vi "MAIN.vi"() -> ()   [LabVIEW 2012]
uses:
  Control/#TD_ThreadsStates.ctl
  Signal/#TD_SignalStorageCommand.ctl
panel:
  in  "Cancel Button":bool
  in  "Results":bool
  in  "Analysis":bool
  in  "Settings":bool
  in  "Signals":bool
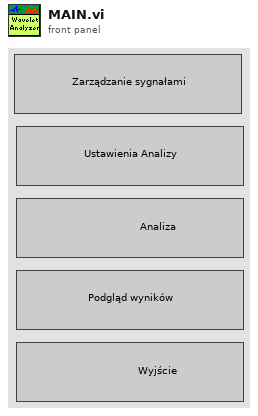
[diagram p1: front panel]
types:
  T1 = typedef "#TD_ThreadsStates.ctl" = cluster{"SigMgmntActive?":bool, "ResltVivActive?":bool, "SettngsMngActive?":bool}
  T2 = typedef "#TD_SignalStorageCommand.ctl" = enum16{"Reset_Storage", "Add_Signal", "Insert_Signal", "Del_Signal", "Replace_Signal", "Get_Signal", "Get_Signal_List", "Change_Signal_Name", "Change_Signal_Descr"}
  T3 = enum32{"Invalid", "Standard", "Closed", "Hidden", "Minimized", "Maximized"}
  T4 = enum32{"Bad", "Idle", "Run top level", "Running"}
  T5 = typedef "#TD_AnalysisSettings.ctl" = cluster{"DecompLevel":i32, "WaveletsToUse":enum16{"db02", "db03", "db04", "db05", "db06", "db07", "db08", "db09", "db10", "db11", "db12", "db13", "db14", "Haar", "bior1_3", "bior1_5", "bior2_2", "bior2_4", "bior2_6", "bior2_8", "bior3_1", "bior3_3", "bior3_5", "bior3_7", "bior3_9", "bior4_4 (FBI)", "bior5_5", "bior6_8", "coif1", "coif2", "coif3", "coif4", "coif5", "sym2", "sym3", "sym4", "sym5", "sym6", "sym7", "sym8"}[], "SignalToAnalysisNb":i32}
  T6 = enum16{"db02", "db03", "db04", "db05", "db06", "db07", "db08", "db09", "db10", "db11", "db12", "db13", "db14", "Haar", "bior1_3", "bior1_5", "bior2_2", "bior2_4", "bior2_6", "bior2_8", "bior3_1", "bior3_3", "bior3_5", "bior3_7", "bior3_9", "bior4_4 (FBI)", "bior5_5", "bior6_8", "coif1", "coif2", "coif3", "coif4", "coif5", "sym2", "sym3", "sym4", "sym5", "sym6", "sym7", "sym8"}[]
  T7 = typedef "#TD_SignalStorageData.ctl" = cluster{"Signal Name":string, "Signal":waveform(dbl), "Description":string}
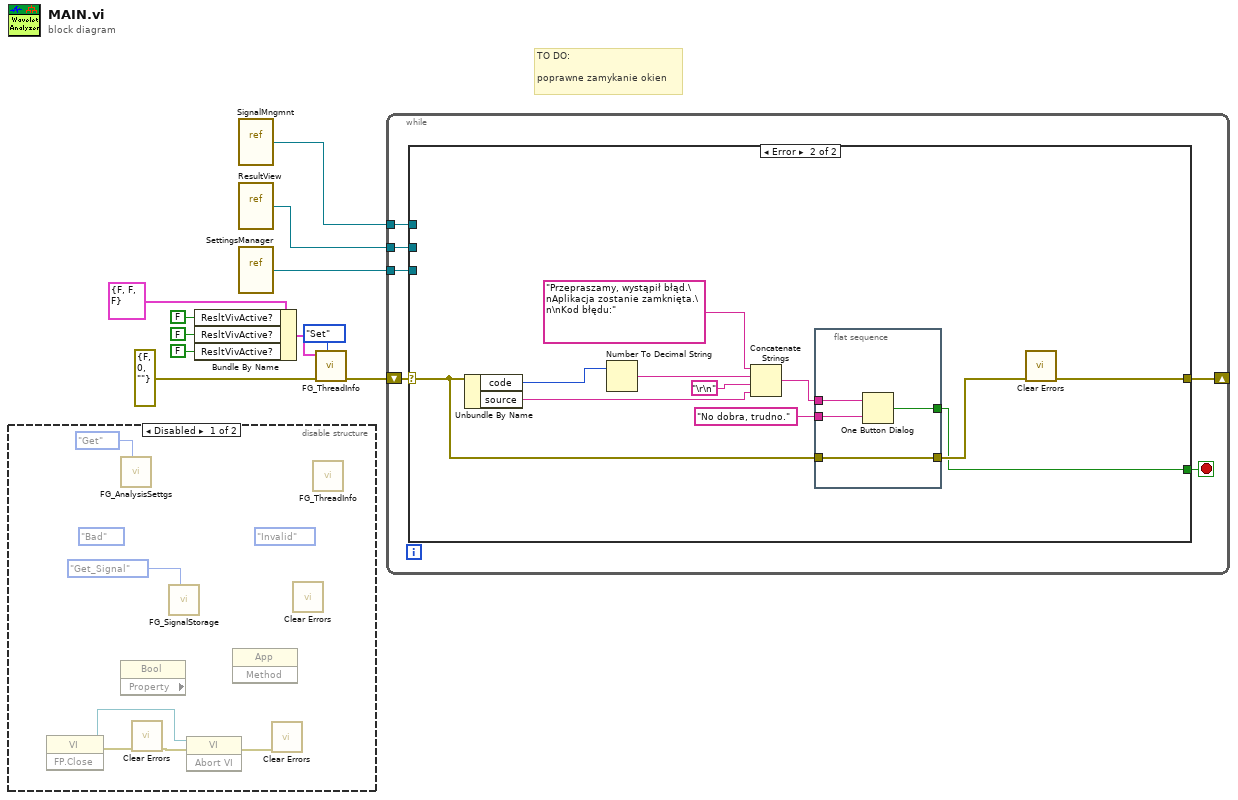
[diagram p0: block diagram]
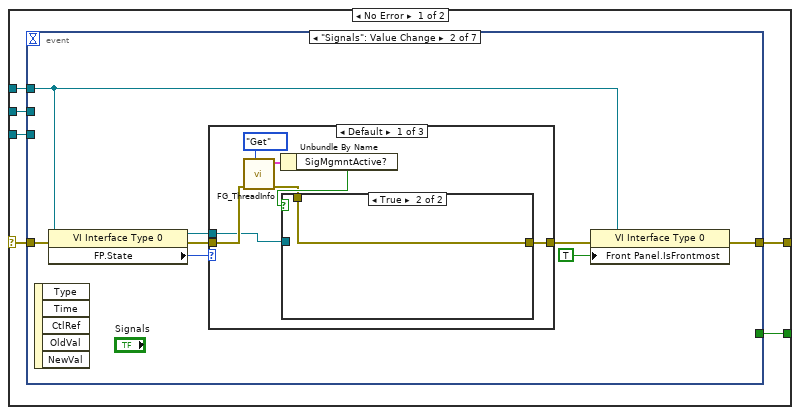
[diagram p3: hidden frame]
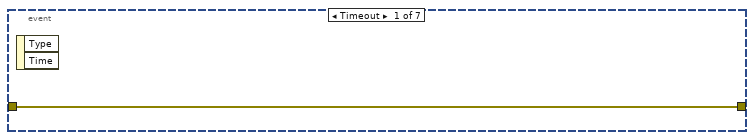
[diagram p4: hidden frame]
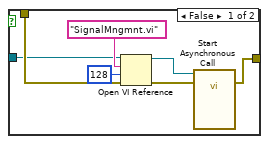
[diagram p5: hidden frame]
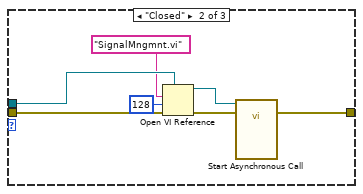
[diagram p6: hidden frame]
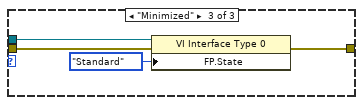
[diagram p7: hidden frame]
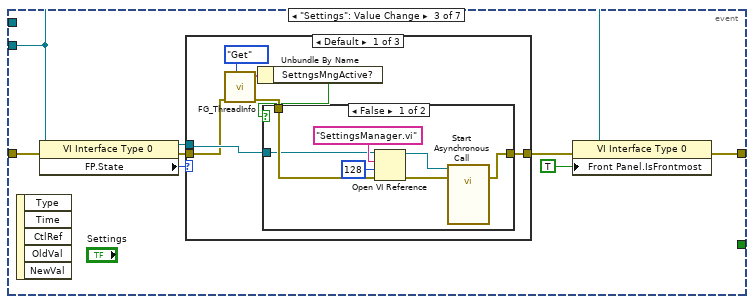
[diagram p8: hidden frame]
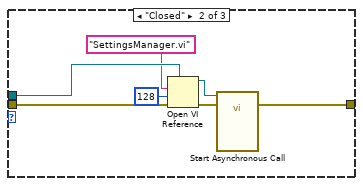
[diagram p10: hidden frame]
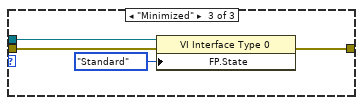
[diagram p11: hidden frame]
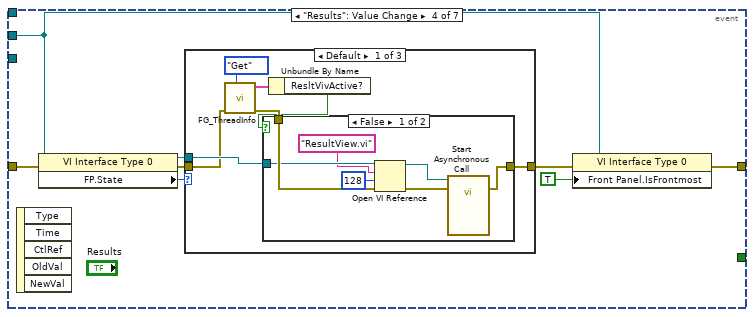
[diagram p12: hidden frame]
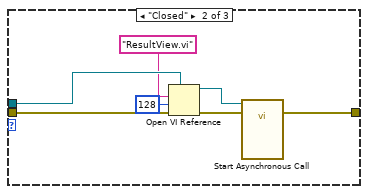
[diagram p14: hidden frame]
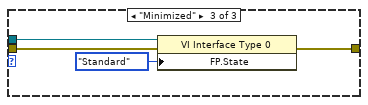
[diagram p15: hidden frame]
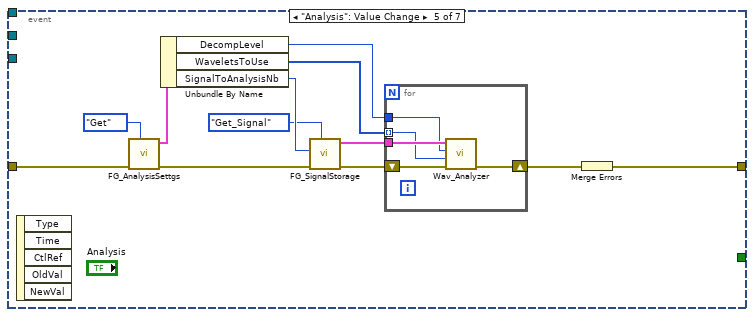
[diagram p16: hidden frame]
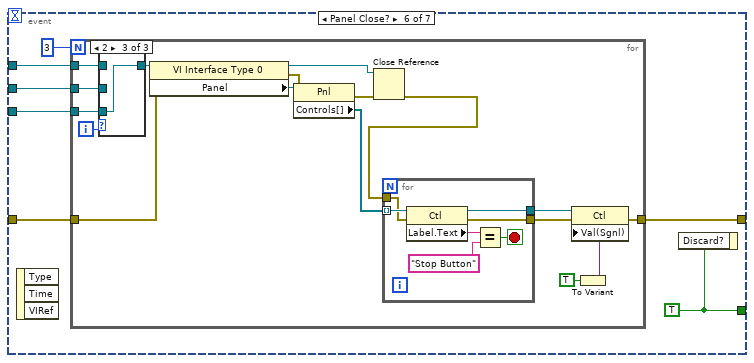
[diagram p17: hidden frame]
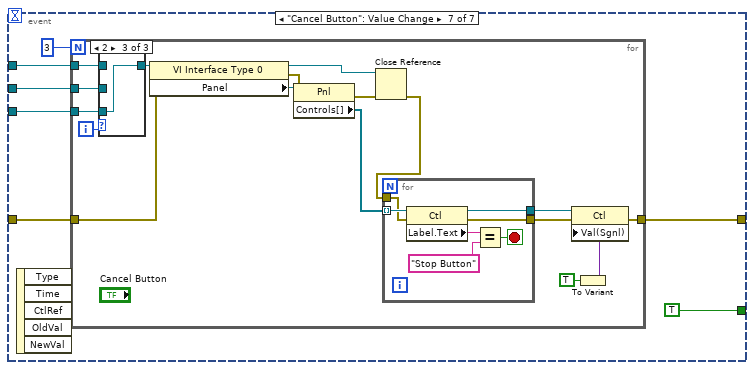
[diagram p20: hidden frame]
diagram:
  # "TO DO:\n\npoprawne zamykanie okien"
  n1 = disable-structure shown="Disabled" {
    frame Disabled {
      (unwired) T3."Invalid" ("Front Panel Window:State")
      (unwired) T4."Bad" ("Execution:State")
      n2 = invoke class="VI" method="FP.Close"() -> (reference out=w15:refnum<vi>, error out=w17:errorcluster)  [unwired: 3 in, 1 out]
      n3 = call "FG_AnalysisSettgs.vi"("Command"=enum16{"Set", "Get", "Reset"}."Get") -> ("error in (no error)"=w19:errorcluster)  [unwired: 8 in, 2 out]
      n4 = property class="Bool" props=[]() -> ()  [unwired: 2 in, 3 out]
      n5 = call <vilib>:"Clear Errors.vi"("error in (no error)"=w17) -> ("error out"=w16:errorcluster)  [unwired: 6 in]
      n6 = call "FG_SignalStorage.vi"("Command"=#TD_SignalStorageCommand."Get_Signal") -> ()  [unwired: 8 in, 3 out]
      n7 = invoke class="VI" method="Abort VI"(reference=w15, error in=w16) -> (reference out=w12:refnum<vi>, error out=w14:errorcluster)  [unwired: 1 in, 1 out]
      n8 = invoke class="App" method=#-1() -> ()  [unwired: 3 in, 3 out]
      n9 = call <vilib>:"Clear Errors.vi"("error in (no error)"=w14) -> ("error out"=w13:errorcluster)  [unwired: 6 in]
      n10 = call <vilib>:"Clear Errors.vi"() -> ()  [unwired: 7 in, 1 out]
      n11 = call "FG_ThreadInfo.vi"() -> ()  [unwired: 10 in, 2 out]
    }
    frame Enabled {
    }
  }
  n12 = Bundle By Name(cluster=T1 {"SigMgmntActive?"=FALSE, "ResltVivActive?"=FALSE, "SettngsMngActive?"=FALSE} ("ThreadsStates Out"), "ResltVivActive?"=FALSE ("SigMgmntActive?"), "ResltVivActive?"=FALSE, "ResltVivActive?"=FALSE) -> (w2:T1)
  n13 = vi-ref "SignalMngmnt.vi"() -> (w11:refnum<vi>)
  n14 = vi-ref "ResultView.vi"() -> (w10:refnum<vi>)
  n15 = vi-ref "SettingsManager.vi"() -> (w9:refnum<vi>)
  n16 = call "FG_ThreadInfo.vi"("Command"=enum16{"Set", "Get"}."Set", "error in (no error)"=errorcluster {"status"=FALSE, "code"=0, "source"=""} ("error constant"), "ThreadsStates"=w2) -> ("error out"=w6:errorcluster)  [unwired: 7 in, 1 out]
  n17 = while {
    shift-right: [w25] -> _
    shift-left: w6 -> [w24]
    tunnel: w11 -> [w23]
    tunnel: w10 -> [w22]
    tunnel: w9 -> [w21]
    stop <- w26 stop-if-true
    n18 = case shown="Error" w24 {
      selector: w24 -> [w30 w224]
      tunnel: [w32 w222] -> w26
      tunnel: [w31 w221] -> w25
      tunnel: w23 -> [w29 _]
      tunnel: w22 -> [w28 _]
      tunnel: w21 -> [w27 _]
      frame No Error {
        n19 = event shown="[1] \"Signals\": Value Change" {
          selector: _ -> [_ _ _ _ _ _ _]
          dyn-events: _ -> [_ _ _ _ _ _ _]
          timeout: _ -> [_ _ _ _ _ _ _]
          tunnel: [_ _ _ _ _ w159 TRUE] -> w32
          tunnel: [w33 w36 w70 w104 w136 w153 w187] -> w31
          tunnel: w30 -> [w33 w40 w74 w108 w147 w154 w188]
          tunnel: w29 -> [_ w35 _ _ _ w157 w191]
          tunnel: w28 -> [_ _ _ w102 _ w156 w190]
          tunnel: w27 -> [_ _ w68 _ _ w155 w189]
          event Timeout {
            n20 = event-data() -> ()  [unwired: 1 in, 2 out]
          }
          event "Signals": Value Change {
            n21 = event-data() -> ()  [unwired: 1 in, 5 out]
            n22 = property class="VI Interface Type 0"(reference=w35, error in=w40) -> (reference out=w41:refnum<vi>, error out=w38:errorcluster, "FP.State"=w39:T3)
            n23 = case shown="Default" w39 {
              tunnel: w41 -> [w43 w63 w66]
              tunnel: w38 -> [w48 w59 w67]
              tunnel: [w42 w57 w64] -> w37
              frame Default {
                n24 = call "FG_ThreadInfo.vi"("Command"=enum16{"Set", "Get"}."Get", "error in (no error)"=w48) -> ("error out"=w44:errorcluster, "ThreadsStates Out"=w46:T1)  [unwired: 8 in]
                n25 = Unbundle By Name(w46) -> ("SigMgmntActive?"=w45:bool)
                n26 = case shown="True" w45 {
                  tunnel: w44 -> [w51 w56]
                  tunnel: w43 -> [w50 _]
                  tunnel: [w49 w56] -> w42
                  frame False {
                    n27 = Open VI Reference(type specifier VI Refnum (for type only)=w50, vi path="SignalMngmnt.vi" ("name or relative path"), options=128, error in (no error)=w51) -> (vi reference=w52:refnum<vi>, error out=w55:errorcluster)  [unwired: 2 in]
                    n28 = call-by-ref "Start Asynchronous Call"(reference=w52, error in=w55) -> (error out=w49:errorcluster)  [unwired: 11 in, 2 out]
                  }
                  frame True {
                  }
                }
              }
              frame "Closed" {
                n29 = Open VI Reference(type specifier VI Refnum (for type only)=w63, vi path="SignalMngmnt.vi" ("name or relative path"), options=128, error in (no error)=w59) -> (vi reference=w62:refnum<vi>, error out=w58:errorcluster)  [unwired: 2 in]
                n30 = call-by-ref "Start Asynchronous Call"(reference=w62, error in=w58) -> (error out=w57:errorcluster)  [unwired: 11 in, 2 out]
              }
              frame "Minimized" {
                n31 = property class="VI Interface Type 0"(reference=w66, error in=w67, "FP.State"=T3."Standard" ("Front Panel Window:State")) -> (error out=w64:errorcluster)  [unwired: 1 out]
              }
            }
            n32 = property class="VI Interface Type 0"(reference=w35, error in=w37, "Front Panel.IsFrontmost"=TRUE ("Front Panel Window:Is Frontmost")) -> (error out=w36:errorcluster)  [unwired: 1 out]
          }
          event "Settings": Value Change {
            n33 = event-data() -> ()  [unwired: 1 in, 5 out]
            n34 = property class="VI Interface Type 0"(reference=w68, error in=w74) -> (reference out=w75:refnum<vi>, error out=w72:errorcluster, "FP.State"=w73:T3)
            n35 = case shown="Default" w73 {
              tunnel: w75 -> [w78 w97 w100]
              tunnel: w72 -> [w77 w96 w101]
              tunnel: [w76 w95 w98] -> w71
              frame Default {
                n36 = call "FG_ThreadInfo.vi"("Command"=enum16{"Set", "Get"}."Get", "error in (no error)"=w77) -> ("error out"=w82:errorcluster, "ThreadsStates Out"=w80:T1)  [unwired: 8 in]
                n37 = Unbundle By Name(w80) -> ("SettngsMngActive?"=w81:bool)
                n38 = case shown="False" w81 {
                  tunnel: w82 -> [w85 w90]
                  tunnel: w78 -> [w84 _]
                  tunnel: [w83 w90] -> w76
                  frame False {
                    n39 = Open VI Reference(type specifier VI Refnum (for type only)=w84, vi path="SettingsManager.vi" ("name or relative path"), options=128, error in (no error)=w85) -> (vi reference=w86:refnum<vi>, error out=w89:errorcluster)  [unwired: 2 in]
                    n40 = call-by-ref "Start Asynchronous Call"(reference=w86, error in=w89) -> (error out=w83:errorcluster)  [unwired: 11 in, 2 out]
                  }
                  frame True {
                  }
                }
              }
              frame "Closed" {
                n41 = Open VI Reference(type specifier VI Refnum (for type only)=w97, vi path="SettingsManager.vi" ("name or relative path"), options=128, error in (no error)=w96) -> (vi reference=w94:refnum<vi>, error out=w91:errorcluster)  [unwired: 2 in]
                n42 = call-by-ref "Start Asynchronous Call"(reference=w94, error in=w91) -> (error out=w95:errorcluster)  [unwired: 11 in, 2 out]
              }
              frame "Minimized" {
                n43 = property class="VI Interface Type 0"(reference=w100, error in=w101, "FP.State"=T3."Standard" ("Front Panel Window:State")) -> (error out=w98:errorcluster)  [unwired: 1 out]
              }
            }
            n44 = property class="VI Interface Type 0"(reference=w68, error in=w71, "Front Panel.IsFrontmost"=TRUE ("Front Panel Window:Is Frontmost")) -> (error out=w70:errorcluster)  [unwired: 1 out]
          }
          event "Results": Value Change {
            n45 = event-data() -> ()  [unwired: 1 in, 5 out]
            n46 = property class="VI Interface Type 0"(reference=w102, error in=w108) -> (reference out=w109:refnum<vi>, error out=w106:errorcluster, "FP.State"=w107:T3)
            n47 = case shown="Default" w107 {
              tunnel: w109 -> [w112 w131 w134]
              tunnel: w106 -> [w111 w127 w135]
              tunnel: [w110 w125 w132] -> w105
              frame Default {
                n48 = call "FG_ThreadInfo.vi"("Command"=enum16{"Set", "Get"}."Get", "error in (no error)"=w111) -> ("error out"=w116:errorcluster, "ThreadsStates Out"=w114:T1)  [unwired: 8 in]
                n49 = Unbundle By Name(w114) -> ("ResltVivActive?"=w115:bool)
                n50 = case shown="False" w115 {
                  tunnel: w116 -> [w120 w124]
                  tunnel: w112 -> [w119 _]
                  tunnel: [w118 w124] -> w110
                  frame False {
                    n51 = Open VI Reference(type specifier VI Refnum (for type only)=w119, vi path="ResultView.vi" ("name or relative path"), options=128, error in (no error)=w120) -> (vi reference=w121:refnum<vi>, error out=w123:errorcluster)  [unwired: 2 in]
                    n52 = call-by-ref "Start Asynchronous Call"(reference=w121, error in=w123) -> (error out=w118:errorcluster)  [unwired: 11 in, 2 out]
                  }
                  frame True {
                  }
                }
              }
              frame "Closed" {
                n53 = Open VI Reference(type specifier VI Refnum (for type only)=w131, vi path="ResultView.vi" ("name or relative path"), options=128, error in (no error)=w127) -> (vi reference=w130:refnum<vi>, error out=w126:errorcluster)  [unwired: 2 in]
                n54 = call-by-ref "Start Asynchronous Call"(reference=w130, error in=w126) -> (error out=w125:errorcluster)  [unwired: 11 in, 2 out]
              }
              frame "Minimized" {
                n55 = property class="VI Interface Type 0"(reference=w134, error in=w135, "FP.State"=T3."Standard" ("Front Panel Window:State")) -> (error out=w132:errorcluster)  [unwired: 1 out]
              }
            }
            n56 = property class="VI Interface Type 0"(reference=w102, error in=w105, "Front Panel.IsFrontmost"=TRUE ("Front Panel Window:Is Frontmost")) -> (error out=w104:errorcluster)  [unwired: 1 out]
          }
          event "Analysis": Value Change {
            n57 = event-data() -> ()  [unwired: 1 in, 5 out]
            n58 = call "FG_AnalysisSettgs.vi"("Command"=enum16{"Set", "Get", "Reset"}."Get", "error in (no error)"=w147) -> ("error out"=w146:errorcluster, "Settings Out"=w141:T5)  [unwired: 8 in]
            n59 = Unbundle By Name(w141) -> ("DecompLevel"=w137:i32, "WaveletsToUse"=w138:T6, "SignalToAnalysisNb"=w140:i32)
            n60 = call "FG_SignalStorage.vi"("Command"=#TD_SignalStorageCommand."Get_Signal", "error in (no error)"=w146, "SignalNumber"=w140) -> ("error out"=w145:errorcluster, "DataOut"=w142:T7)  [unwired: 6 in, 1 out]
            n61 = for {
              tunnel: w142 -> [w150]
              tunnel: w138 -> [w149] mode=indexing
              tunnel: w137 -> [w148]
              shift-right: [w151] -> w144
              shift-left: w145 -> [w152]
              n62 = call "Wav_Analyzer.vi"("error in (no error)"=w152, "Wavelet"=w149, "Decomposition Level"=w148, "DataIn"=w150) -> ("error out"=w151:errorcluster)  [unwired: 7 in]
            }
            n63 = Merge Errors(w144) -> (w136:errorcluster)
          }
          event Panel Close? {
            w159 = TRUE
            n64 = event-data() -> ()  [unwired: 1 in, 3 out]
            n65 = for {
              N: 3 -> [_]
              tunnel: w157 -> [w174]
              tunnel: w156 -> [w173]
              tunnel: w155 -> [w172]
              tunnel: w154 -> [w169]
              tunnel: [w163] -> w153
              i -> [w175]
              n66 = case shown="2" w175 {
                tunnel: [w184 w185 w186] -> w171
                tunnel: w174 -> [w184 _ _]
                tunnel: w173 -> [_ w185 _]
                tunnel: w172 -> [_ _ w186]
                frame 0, Default {
                }
                frame 1 {
                }
                frame 2 {
                }
              }
              n67 = property class="VI Interface Type 0"(reference=w171, error in=w169) -> (reference out=w160:refnum<vi>, error out=w176:errorcluster, "Panel"=w170:refnum<vi>)
              n68 = property class="Pnl"(reference=w170, error in=w176) -> (error out=w162:errorcluster, "Controls[]"=w168:refnum<vi>[])  [unwired: 1 out]
              n69 = Close Reference(reference=w160, error in (no error)=w162) -> (error out=w161:errorcluster)
              n70 = for {
                tunnel: w168 -> [w183] mode=indexing
                tunnel: w161 -> [w182]
                tunnel: [w178] -> w167
                tunnel: [w177] -> w166
                stop <- w179 stop-if-true
                n71 = property class="Ctl"(reference=w183, error in=w182) -> (reference out=w178:refnum<vi>, error out=w177:errorcluster, "Label.Text"=w181:string)
                n72 = Equal?(x=w181, y="Stop Button") -> (x = y?=w179:bool)
              }
              n73 = To Variant(anything=TRUE) -> (Variant=w164:variant)
              n74 = property class="Ctl"(reference=w167, error in=w166, "Val(Sgnl)"=w164) -> (error out=w163:errorcluster)  [unwired: 1 out]
            }
            n75 = event-data("Discard?"=w159) -> ()  [unwired: 1 in, 1 out]
          }
          event "Cancel Button": Value Change {
            n76 = event-data() -> ()  [unwired: 1 in, 5 out]
            n77 = for {
              N: 3 -> [_]
              tunnel: w191 -> [w208]
              tunnel: w190 -> [w207]
              tunnel: w189 -> [w206]
              tunnel: w188 -> [w203]
              tunnel: [w197] -> w187
              i -> [w209]
              n78 = case shown="2" w209 {
                tunnel: [w218 w219 w220] -> w205
                tunnel: w208 -> [w218 _ _]
                tunnel: w207 -> [_ w219 _]
                tunnel: w206 -> [_ _ w220]
                frame 0, Default {
                }
                frame 1 {
                }
                frame 2 {
                }
              }
              n79 = property class="VI Interface Type 0"(reference=w205, error in=w203) -> (reference out=w196:refnum<vi>, error out=w210:errorcluster, "Panel"=w204:refnum<vi>)
              n80 = property class="Pnl"(reference=w204, error in=w210) -> (error out=w195:errorcluster, "Controls[]"=w202:refnum<vi>[])  [unwired: 1 out]
              n81 = Close Reference(reference=w196, error in (no error)=w195) -> (error out=w194:errorcluster)
              n82 = for {
                tunnel: w202 -> [w217] mode=indexing
                tunnel: w194 -> [w216]
                tunnel: [w212] -> w201
                tunnel: [w211] -> w200
                stop <- w213 stop-if-true
                n83 = property class="Ctl"(reference=w217, error in=w216) -> (reference out=w212:refnum<vi>, error out=w211:errorcluster, "Label.Text"=w215:string)
                n84 = Equal?(x=w215, y="Stop Button") -> (x = y?=w213:bool)
              }
              n85 = To Variant(anything=TRUE) -> (Variant=w198:variant)
              n86 = property class="Ctl"(reference=w201, error in=w200, "Val(Sgnl)"=w198) -> (error out=w197:errorcluster)  [unwired: 1 out]
            }
          }
        }
      }
      frame Error {
        n87 = Unbundle By Name(w224) -> ("code"=w230:i32, "source"=w227:string)
        n88 = Number To Decimal String(number=w230) -> (decimal integer string=w229:string)  [unwired: 1 in]
        n89 = Concatenate Strings("Przepraszamy, wystąpił błąd.\nAplikacja zostanie zamknięta.\n\nKod błędu:", w229, "\r\n", w227) -> (w226:string)
        n90 = flat-sequence {
          tunnel: w226 -> [w235]
          tunnel: "No dobra, trudno." ("button name (\"OK\")") -> [w234]
          tunnel: [w233] -> w222
          tunnel: w224 -> [w232]
          tunnel: [w232] -> w223
          frame #0 {
            n91 = One Button Dialog(message=w235, button name ("OK")=w234) -> (true=w233:bool)
          }
        }
        n92 = call <vilib>:"Clear Errors.vi"("error in (no error)"=w223) -> ("error out"=w221:errorcluster)  [unwired: 6 in]
      }
    }
  }
